vi "Add light-dark measurements to queue.vi"(9 "Measuring all pixels on cell?":bool, 10 "Scan settings array":T3[](array[typedef]) {"J-t Illumination conditions" items=["Light only", "Dark only", "Light then dark", "Dark then light"]; "No. of scan rate steps" min=1.0 step=1.0; "Illumination conditions" items=["Light only", "Dark only", "Light then dark", "Dark then light", "Light then dark then light", "Dark then light then dark"]; "Time Constant (s)" items=["0.01s", "0.03s", "0.1s", "0.3s", "1s", "3s"]; "Only repeat for best pixel" items=["only for best pixel", "for best 2 pixels", "for best 3 pixels", "for best 4 pixels", "for best 5 pixels", "for best 6 pixels", "for best 7 pixels", "for all pixels"]; "No. of repeat scans" min=1.0 step=1.0; "EQE best pixel only" items=["only the best pixel", "the best 2 pixel", "the best 3 pixel", "the best 4 pixel", "the best 5 pixel", "the best 6 pixel", "the best 7 pixel", "all pixels"]; "P dep best pixel only" items=["only the best pixel", "the best 2 pixels", "the best 3 pixels", "the best 4 pixels", "the best 5 pixels", "the best 6 pixels", "the best 7 pixels", "all pixels"]; "Max power best pixel only" items=["only the best pixel", "the best 2 pixels", "the best 3 pixels", "the best 4 pixels", "the best 5 pixels", "the best 6 pixels", "the best 7 pixels", "all pixels"]; "J-t best pixel only" items=["only the best pixel", "the best 2 pixels", "the best 3 pixels", "the best 4 pixels", "the best 5 pixels", "the best 6 pixels", "the best 7 pixels", "all pixels"]; "Integration time" items=["Fast", "Normal", "High Accuracy"]; "Stabilisation mode" items=["V", "I"]; "Measurement delay (ms)" min=10.0}, 11 "Cell settings cluster":T2) -> (3 "Light/dark array":T1(array[cluster]))   [LabVIEW 2011]
uses:
  TypeDefs/Scan settings.ctl
  TypeDefs/Settings Boolean.ctl
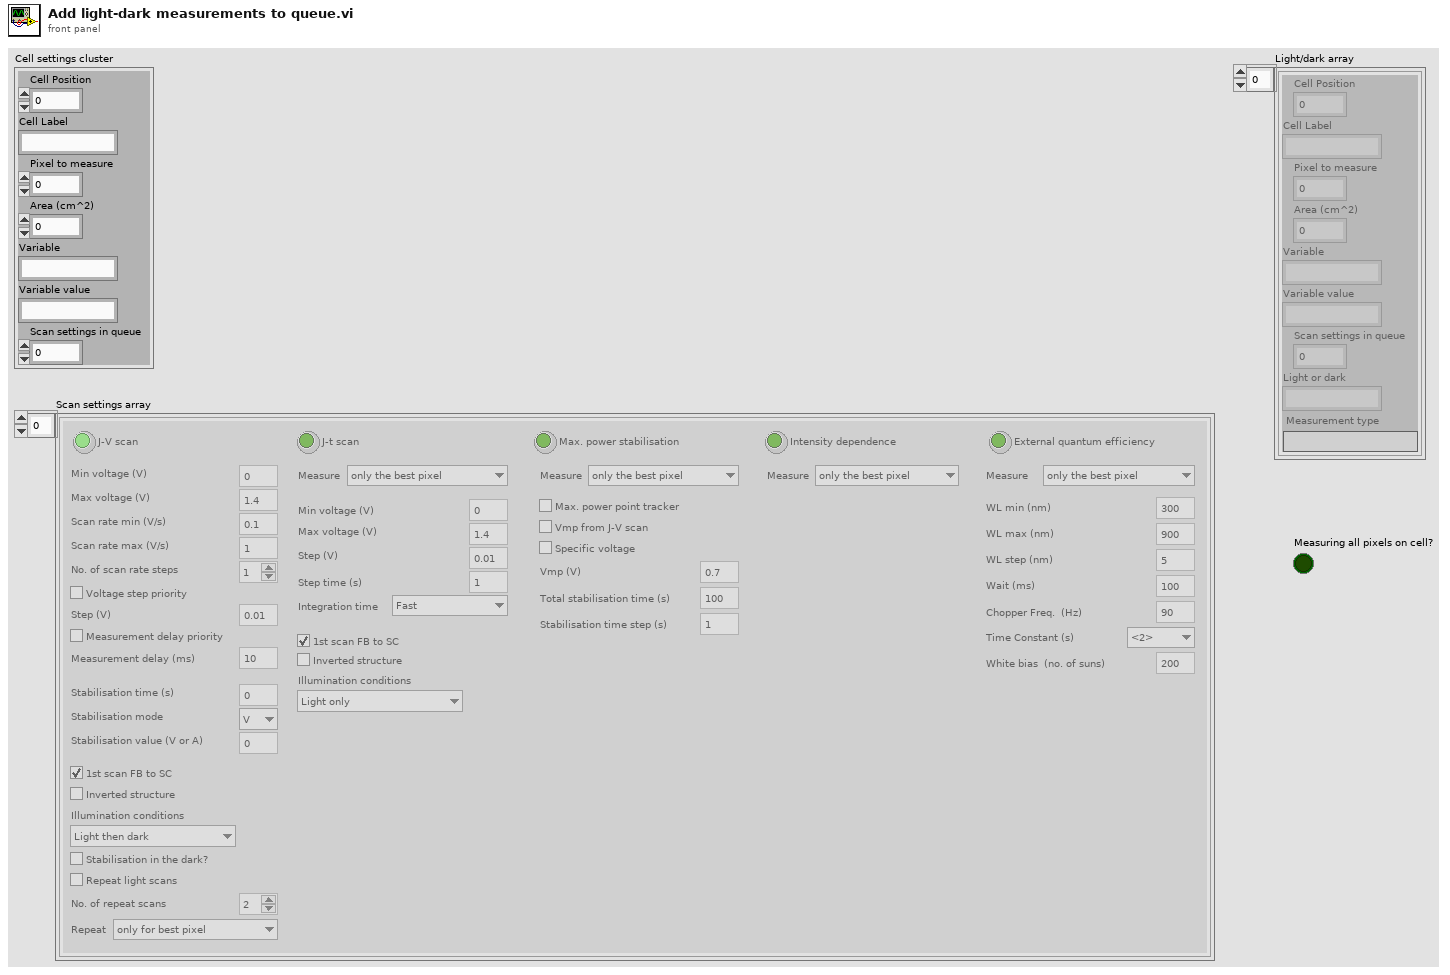
[diagram p1: front panel]
types:
  T1 = cluster{"Cell Position":i32, "Cell Label":string, "Pixel to measure":u16, "Area (cm^2)":dbl, "Variable":string, "Variable value":string, "Scan settings in queue":u16, "Light or dark":string, "Measurement type":string}[]
  T2 = cluster{"Cell Position":i32, "Cell Label":string, "Pixel to measure":u16, "Area (cm^2)":dbl, "Variable":string, "Variable value":string, "Scan settings in queue":u16}
  T3 = typedef "Scan settings.ctl" = cluster{"J-V scan":T4, "J-t scan":bool, "Min voltage (V)":dbl, "Max voltage (V)":dbl, "Step (V)":dbl, "Measurement delay (ms)":dbl, "1st scan FB-SC":bool, "Inverted structure":bool, "Stabilisation time (s)":dbl, "Stabilisation mode":u16, "Stabilisation value (V or A) ":dbl, "Step time (s)":dbl, "Integration time":u16, "Repeat light scans":bool, "Stabilisation in the dark?":bool, "J-t Min (V)":dbl, "J-t Max (V)":dbl, "J-t Step (V)":dbl, "Max. power stabilisation":bool, "J-t 1st scan FB-SC":bool, "J-t Inverted structure":bool, "Max power tracking":bool, "Vmp (V)":dbl, "Total stabilisation time (s)":dbl, "J-t best pixel only":u16, "Max power best pixel only":u16, "Vmp from J-V scan":bool, "Intensity dependence":bool, "P dep best pixel only":u16, "External quantum efficiency":bool, "EQE best pixel only":u16, "WL min (nm)":dbl, "WL max (nm)":dbl, "WL step (nm)":dbl, "Wait (ms)":dbl, "No. of repeat scans":dbl, "Only repeat for best pixel":u16, "Chopper Freq.  (Hz)":dbl, "Time Constant (s)":dbl, "Stabilisation time step (s)":dbl, "Illumination conditions":u16, "Scan rate min (V/s)":dbl, "Scan rate max (V/s)":dbl, "No. of scan rate steps":dbl, "Scan rate voltage step priority":bool, "Scan rate measurement delay priority":bool, "J-t Illumination conditions":u16, "White bias  (no. of suns)":dbl, "Max P stab. Specific voltage":bool}
  T4 = typedef "Settings Boolean.ctl" = bool
  T5 = cluster{"Cell Position":i32, "Cell Label":string, "Pixel to measure":u16, "Area (cm^2)":dbl, "Variable":string, "Variable value":string, "Scan settings in queue":u16, "Light or dark":string, "Measurement type":string}
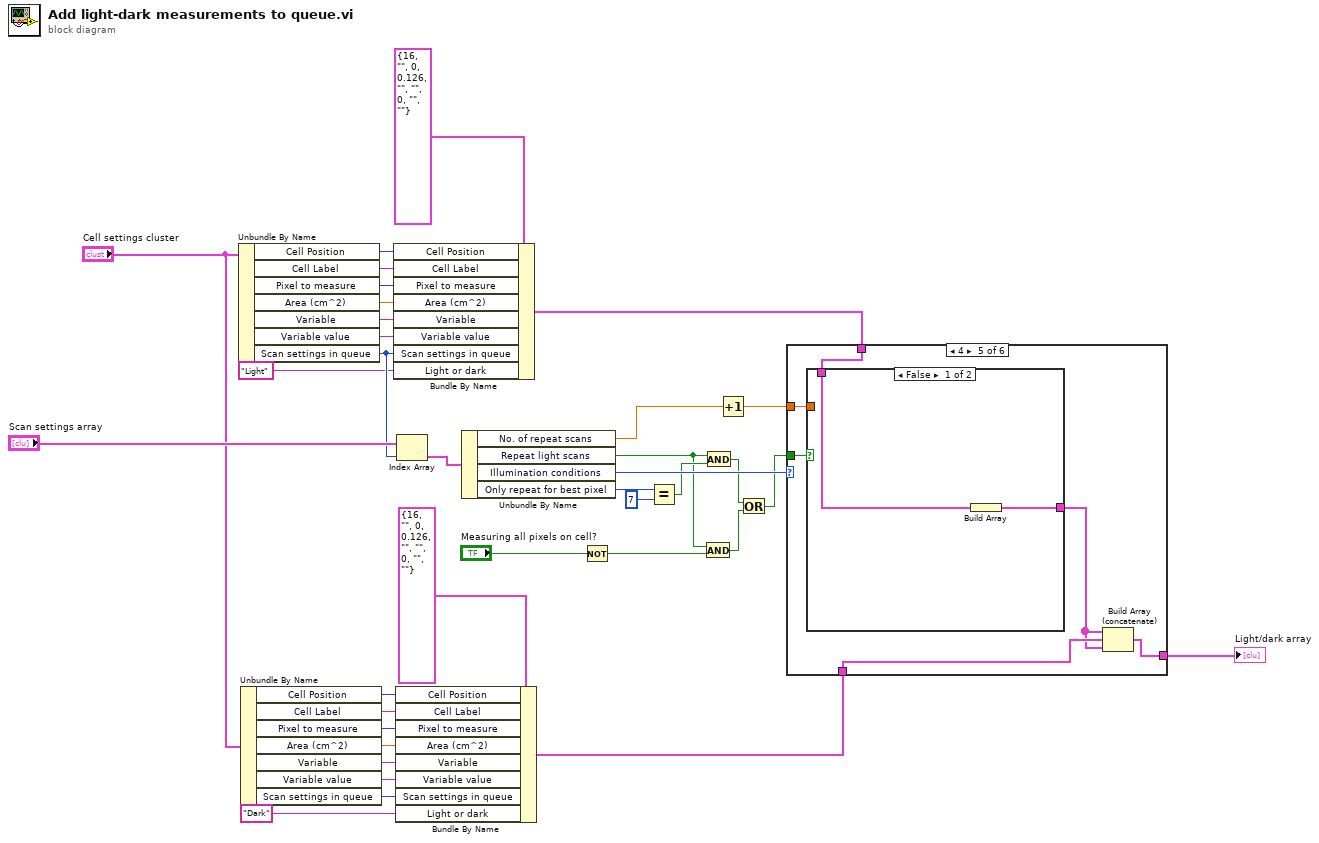
[diagram p0: block diagram]
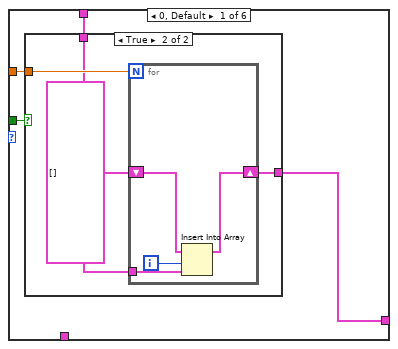
[diagram p2: hidden frame]
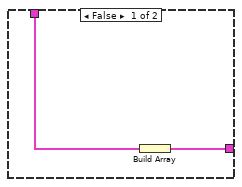
[diagram p3: hidden frame]
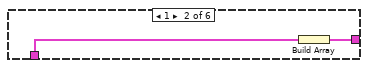
[diagram p4: hidden frame]
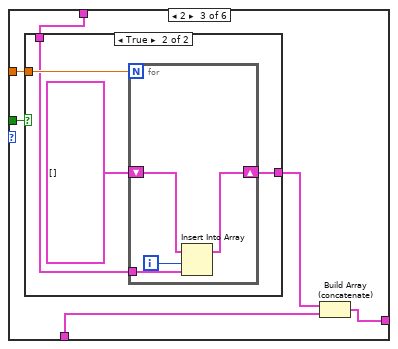
[diagram p5: hidden frame]
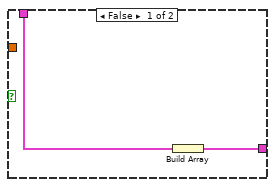
[diagram p6: hidden frame]
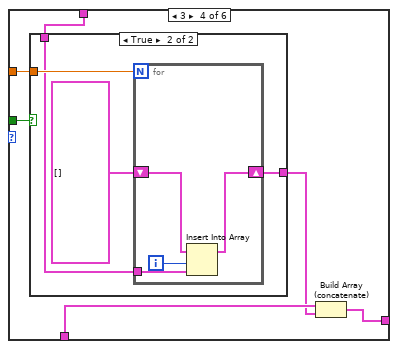
[diagram p7: hidden frame]
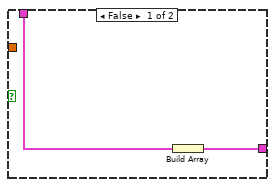
[diagram p8: hidden frame]
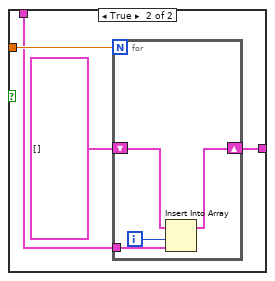
[diagram p9: hidden frame]
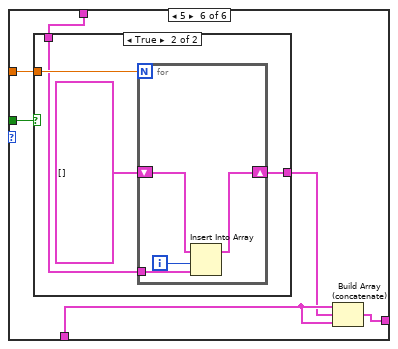
[diagram p10: hidden frame]
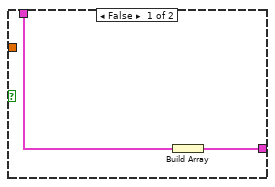
[diagram p11: hidden frame]
diagram:
  n1 = Unbundle By Name("Cell settings cluster") -> ("Cell Position"=w16:i32, "Cell Label"=w17:string, "Pixel to measure"=w18:u16, "Area (cm^2)"=w19:dbl, "Variable"=w20:string, "Variable value"=w21:string, "Scan settings in queue"=w34:u16)
  n2 = Unbundle By Name("Cell settings cluster") -> ("Cell Position"=w23:i32, "Cell Label"=w24:string, "Pixel to measure"=w25:u16, "Area (cm^2)"=w26:dbl, "Variable"=w27:string, "Variable value"=w28:string, "Scan settings in queue"=w29:u16)
  n3 = Bundle By Name(cluster=T5 {"Cell Position"=16, "Cell Label"="", "Pixel to measure"=0, "Area (cm^2)"=0.126, "Variable"="", "Variable value"="", "Scan settings in queue"=0, "Light or dark"="", "Measurement type"=""} ("System Cluster"), "Cell Position"=w16, "Cell Label"=w17, "Pixel to measure"=w18, "Area (cm^2)"=w19, "Variable"=w20, "Variable value"=w21, "Scan settings in queue"=w34, "Light or dark"="Light") -> (w14:T5)
  n4 = Bundle By Name(cluster=T5 {"Cell Position"=16, "Cell Label"="", "Pixel to measure"=0, "Area (cm^2)"=0.126, "Variable"="", "Variable value"="", "Scan settings in queue"=0, "Light or dark"="", "Measurement type"=""} ("System Cluster"), "Cell Position"=w23, "Cell Label"=w24, "Pixel to measure"=w25, "Area (cm^2)"=w26, "Variable"=w27, "Variable value"=w28, "Scan settings in queue"=w29, "Light or dark"="Dark") -> (w31:T5)
  n5 = Index Array(array="Scan settings array", index=w34) -> (element=w36:T3)
  n6 = Unbundle By Name(w36) -> ("No. of repeat scans"=w1:dbl, "Repeat light scans"=w8:bool, "Illumination conditions"=w12:u16, "Only repeat for best pixel"=w11:u16)
  n7 = Not(x="Measuring all pixels on cell?") -> (.not. x?=w3:bool)
  n8 = Equal?(x=w11, y=u16 7) -> (x = y?=w9:bool)
  n9 = And(x=w8, y=w3) -> (x .and. y?=w7:bool)
  n10 = And(x=w8, y=w9) -> (x .and. y?=w6:bool)
  n11 = Increment(x=w1) -> (x+1=w2:dbl)
  n12 = Or(x=w6, y=w7) -> (x .or. y?=w5:bool)
  n13 = case shown="4" w12 {
    tunnel: w14 -> [w38 _ w58 w72 w89 w104]
    tunnel: w31 -> [_ w52 w54 w74 w87 w102]
    tunnel: [w37 w51 w53 w73 w85 w103] -> w32
    tunnel: w5 -> [w39 _ w56 w70 w88 w105]
    tunnel: w2 -> [w40 _ w57 w71 w90 w106]
    frame 0, Default {
      n14 = case shown="True" w39 {
        tunnel: w40 -> [_ w46]
        tunnel: w38 -> [w42 w45]
        tunnel: [w41 w43] -> w37
        frame False {
          n15 = Build Array(w42) -> (w41:T1)
        }
        frame True {
          n16 = for {
            N: w46 -> [_]
            tunnel: w45 -> [w49]
            shift-right: [w47] -> w43
            shift-left: T1 [] ("Light/dark array") -> [w48]
            i -> [w50]
            n17 = Insert Into Array(array=w48, index=w50, new element=w49) -> (w47:T1)
          }
        }
      }
    }
    frame 1 {
      n18 = Build Array(w52) -> (w51:T1)
    }
    frame 2 {
      n19 = case shown="True" w56 {
        tunnel: w57 -> [_ w64]
        tunnel: w58 -> [w60 w63]
        tunnel: [w59 w61] -> w55
        frame False {
          n20 = Build Array(w60) -> (w59:T1)
        }
        frame True {
          n21 = for {
            N: w64 -> [_]
            tunnel: w63 -> [w67]
            shift-right: [w65] -> w61
            shift-left: T1 [] ("Light/dark array") -> [w66]
            i -> [w68]
            n22 = Insert Into Array(array=w66, index=w68, new element=w67) -> (w65:T1)
          }
        }
      }
      n23 = Build Array (concatenate)(w55, w54) -> (w53:T1)
    }
    frame 3 {
      n24 = case shown="True" w70 {
        tunnel: w71 -> [_ w80]
        tunnel: w72 -> [w76 w79]
        tunnel: [w75 w77] -> w69
        frame False {
          n25 = Build Array(w76) -> (w75:T1)
        }
        frame True {
          n26 = for {
            N: w80 -> [_]
            tunnel: w79 -> [w83]
            shift-right: [w81] -> w77
            shift-left: T1 [] ("Light/dark array") -> [w82]
            i -> [w84]
            n27 = Insert Into Array(array=w82, index=w84, new element=w83) -> (w81:T1)
          }
        }
      }
      n28 = Build Array (concatenate)(w74, w69) -> (w73:T1)
    }
    frame 4 {
      n29 = case shown="False" w88 {
        tunnel: w90 -> [_ w96]
        tunnel: w89 -> [w92 w95]
        tunnel: [w91 w93] -> w86
        frame False {
          n30 = Build Array(w92) -> (w91:T1)
        }
        frame True {
          n31 = for {
            N: w96 -> [_]
            tunnel: w95 -> [w99]
            shift-right: [w97] -> w93
            shift-left: T1 [] ("Light/dark array") -> [w98]
            i -> [w100]
            n32 = Insert Into Array(array=w98, index=w100, new element=w99) -> (w97:T1)
          }
        }
      }
      n33 = Build Array (concatenate)(w86, w87, w86) -> (w85:T1)
    }
    frame 5 {
      n34 = case shown="True" w105 {
        tunnel: w106 -> [_ w112]
        tunnel: w104 -> [w108 w111]
        tunnel: [w107 w109] -> w101
        frame False {
          n35 = Build Array(w108) -> (w107:T1)
        }
        frame True {
          n36 = for {
            N: w112 -> [_]
            tunnel: w111 -> [w115]
            shift-right: [w113] -> w109
            shift-left: T1 [] ("Light/dark array") -> [w114]
            i -> [w116]
            n37 = Insert Into Array(array=w114, index=w116, new element=w115) -> (w113:T1)
          }
        }
      }
      n38 = Build Array (concatenate)(w102, w101, w102) -> (w103:T1)
    }
  }
  "Light/dark array" <- w32
